vi "Sound_LV_Python.vi"() -> ()   [LabVIEW 2024]
uses:
  <vilib>/Python/Open Venv Python Session.vi
panel:
  out "Tab Control":enum32{"Idle", "Alarm Editor", "Anasayfa"}(tab)
  in  "Start Asistant":bool
  out "Text":string
  # "ALARM"
  # "HOME PAGE"
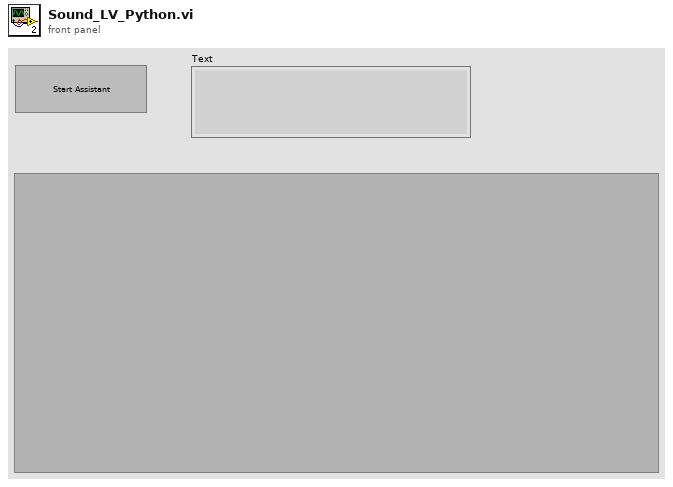
[diagram p1: front panel]
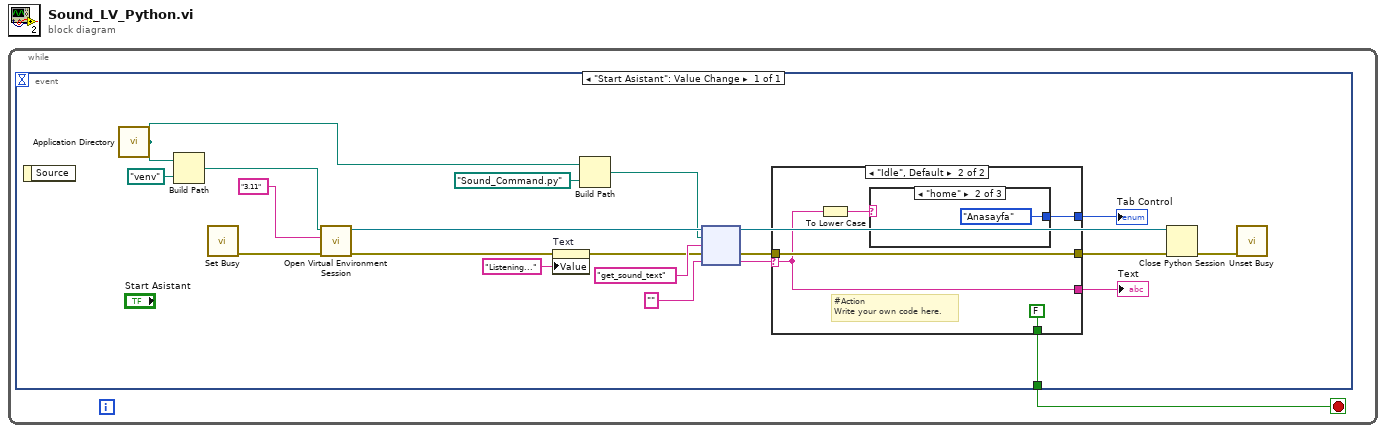
[diagram p0: block diagram]
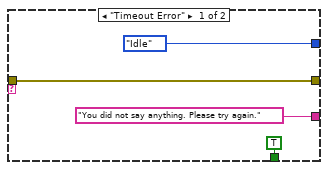
[diagram p2: hidden frame]
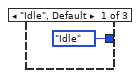
[diagram p3: hidden frame]
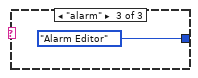
[diagram p4: hidden frame]
diagram:
  n1 = while {
    stop <- w1 stop-if-true
    n2 = event shown="[0] \"Start Asistant\": Value Change" {
      selector: _ -> [_]
      dyn-events: _ -> [_]
      timeout: _ -> [_]
      tunnel: [w11] -> w1
      event "Start Asistant": Value Change {
        n3 = event-data() -> ()  [unwired: 1 in, 1 out]
        n4 = call <vilib>:"Application Directory.vi"() -> ("Application Directory"=w5:path)
        n5 = Build Path(base path=w5, name or relative path=path "venv") -> (appended path=w2:path)
        n6 = call <vilib>:"Set Busy.vi"() -> ("error out"=w7:errorcluster)  [unwired: 10 in, 1 out]
        n7 = call-poly <vilib>:"Open Virtual Environment Session.vi"("error in (no error)"=w7, "Python version"="3.11", "Env path"=w2) -> ("error out"=w10:errorcluster, "session out"=w22:refnum<k35>)  [unwired: 7 in]
        n8 = property on="Text" class="Str"(error in=w10, "Value"="Listening..." ("Text")) -> (error out=w9:errorcluster)  [unwired: 1 in, 1 out]
        n9 = Build Path(base path=w5, name or relative path=path "Sound_Command.py") -> (appended path=w4:path)
        n10 = node(w22, w4, "get_sound_text" ("function name"), w9, "") -> (w21:refnum<k35>, w15:errorcluster, w16:string)  [unwired: 2 out]
        n11 = case shown="\"Idle\", Default" w16 {
          selector: w16 -> [_ w30]
          tunnel: w15 -> [w26 w31]
          tunnel: [w26 w31] -> w14
          tunnel: ["You did not say anything. Please try again." w30] -> w13
          tunnel: [enum32{"Idle", "Alarm Editor", "Anasayfa"}."Idle" ("Tab Control") w28] -> w12
          tunnel: [TRUE FALSE] -> w11
          frame "Timeout Error" {
          }
          frame "Idle", Default {
            # "#Action\nWrite your own code here."
            n12 = To Lower Case(string=w30) -> (all lower case string=w29:string)
            n13 = case shown="\"home\"" w29 {
              tunnel: [enum32{"Idle", "Alarm Editor", "Anasayfa"}."Idle" ("Tab Control") enum32{"Idle", "Alarm Editor", "Anasayfa"}."Anasayfa" ("Tab Control") enum32{"Idle", "Alarm Editor", "Anasayfa"}."Alarm Editor" ("Tab Control")] -> w28
              frame "Idle", Default {
              }
              frame "home" {
              }
              frame "alarm" {
              }
            }
          }
        }
        "Text" <- w13
        "Tab Control" <- w12
        n14 = Close Python Session(session in=w21, error in=w14) -> (11:w18:errorcluster)
        n15 = call <vilib>:"Unset Busy.vi"("error in (no error)"=w18) -> ()  [unwired: 10 in, 1 out]
      }
    }
  }
